vi "get data.vi"(8 "错误输入（无错误）":errorcluster, 11 "VISA GPIB Resource":refnum<visa-resource-name>="GPIB0::2::INSTR" caption="VISA GPIB资源") -> (0 "错误输出":errorcluster, 1 "data":dbl, 2 "Read Buffer":string caption="读取缓冲区", 3 "VISA资源名称输出":refnum<visa-resource-name>)   [LabVIEW 2017]
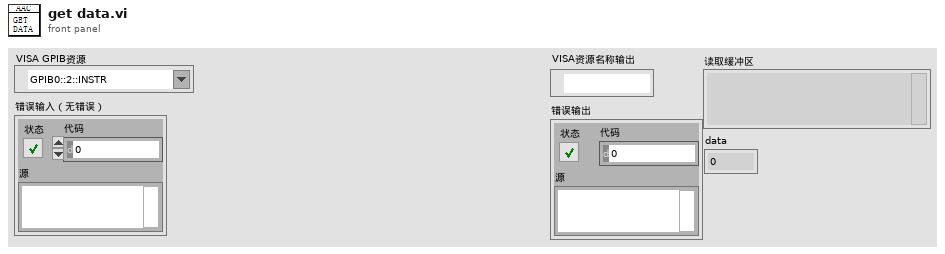
[diagram p1: front panel]
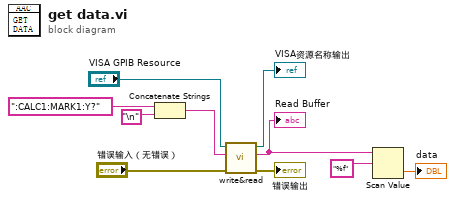
[diagram p0: block diagram]
diagram:
  n1 = Concatenate Strings(":CALC1:MARK1:Y?", "\n") -> (w8:string)
  n2 = call "write&read.vi"("错误输入（无错误）"="错误输入（无错误）", "Write Buffer"=w8, "VISA GPIB Resource"="VISA GPIB Resource") -> ("错误输出"=→"错误输出":errorcluster, "Read Buffer"=w3:string, "VISA资源名称输出"=→"VISA资源名称输出":refnum<visa-resource-name>)  [unwired: 6 in]
  "Read Buffer" <- w3
  n3 = Scan Value(string=w3, format string="%f" ("格式字符串")) -> (value=→"data":dbl)  [unwired: 1 in, 1 out]
